vi "Main.vi"() -> ()   [LabVIEW 2014]
doc: "This template is for the Queued Message Handler design pattern.\n\nThe Event Handling Loop generates messages based on user interface actions.\n\nThe Message Handling Loop processes messages generated by the Event Handling Loop, or by other messages. The messages are string values, so new messages can be added easily to the Message Cases case structure in the Message Handling Loop. Each message cluster can also provide an optional value for Message Data, which is a variant that can be converted to whatever message-specific data is required."
uses:
  support/Type Definitions/UI Data.ctl
  support/Message Queue/Message Queue.lvlib
  Support/User Event - EHL Stop/User Event - EHL Stop.lvlib
  support/Message Queue/Enqueue Message (Single).vi
  <vilib>/ErrorRing/Error Ring.xnode
  Model/Model.lvlib
  DAQ/DAQ.lvlib
  DAQ/TypeDefs/DAQ data.ctl
  PLC/PLC.lvlib
  Logger/Logger.lvlib
  support/Status Logger/Status Log.ctl
  TCP/TCP.lvlib
  TCP/TypeDefs/TCP Data.ctl
  support/Global names.vi
  <vilib>/Utility/error.llb/DialogType.ctl
  <vilib>/Utility/error.llb/Error Cluster From Error Code.vi
  Report/Report.lvlib
  Report/TypeDefs/Report state.ctl
panel:
  out "Power status":bool
  in  "Remote":bool
  in  "Abort":bool
  in  "Stop Line":bool
  in  "Start Line":bool
  out "Status":string
  in  "Tab Control":T1(tab)
  in  "Power switch":bool
  in  "Positon":dbl(slide) scale=0.0..20.0
  in  "Dispose":bool
  in  "Pump":bool
  in  "Flow [l/s]":dbl=10.0
  in  "Potentiometer (AI)":tag
  in  "LED (DO)":tag
  in  "Bistable switch (DI)":tag
  in  "Monostable switch (DI)":tag
  in  "Send":bool
  in  "Message to send":string
  out "Message received":string
  in  "Disconnect":bool
  in  "Connect":bool
  out "Connected?":bool
  in  "Type":enum16{"Server", "Client"}(ring)
  in  "Port":u16
  in  "IP":string
  out "Current machine IP":string
  in  "Current printer":u16(ring) items=["PDFCreator", "OKI DATA CORP C5950 kolor (C-2 218)", "Microsoft XPS Document Writer", "Microsoft Print to PDF", "HP LaserJet Professional P1606dn B&W (M3)", "hp LaserJet 1320 PCL 5 B&W (C-2 307)", "Fax", "Canon MP560 KOLOR (DOM)", "Brother PC-FAX v.3.2", "Brother MFC-L8850CDW KOLOR (M6)", "Brother MFC-L2740DW B&W (M6)", "Brother MFC-L2740DW B&W (M3)", "Brother DCP-9020CDW (Dziekan)"]
  in  "Check printers":bool
  in  "Print report":bool
  in  "TDMS View":bool
  in  "Exit":bool
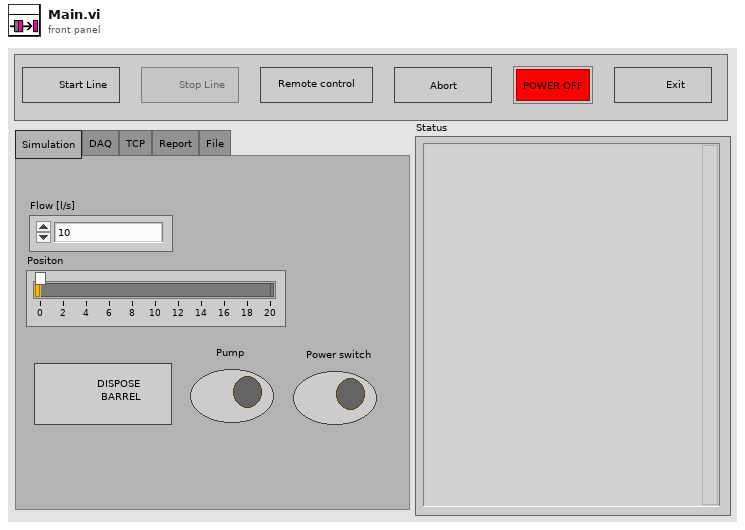
[diagram p1: front panel]
types:
  T1 = enum32{"Simulation", "DAQ", "TCP", "Report", "File"}
  T2 = typedef "Status Log.ctl" = enum16{"Close file", "Open Status file", "Add Status", "Show Status File"}
  T3 = typedef "UI Data.ctl" = cluster{"Start Line Ref":refnum<vi>, "Stop Line Ref":refnum<vi>, "Data Display Ref":refnum<vi>, "Exit Button Ref":refnum<vi>, "Pump Ref":refnum<vi>, "Dispose Ref":refnum<vi>, "Flow Ref":refnum<vi>, "Position Ref":refnum<vi>, "Tab Ref":refnum<vi>, "Print report":refnum<vi>, "Remote":refnum<vi>, "Connection status":refnum<vi>, "Abort":refnum<vi>, "Power status":refnum<vi>, "Power switch":refnum<vi>}
  T4 = typedef "Notifiers.lvlib/Notifiers.ctl" = cluster{"PLC":refnum<notifier>, "Model":refnum<notifier>, "DAQ":refnum<notifier>, "Log":refnum<notifier>, "TCP":refnum<notifier>}
  T5 = typedef "Message Queue.lvlib/All Message Queues.ctl" = cluster{"UI":refnum<queue>, "Model":refnum<queue>, "DAQ":refnum<queue>, "PLC":refnum<queue>, "Log":refnum<queue>, "TCP":refnum<queue>}
  T6 = typedef "Report.lvlib/Report state.ctl" = enum16{"Create report", "Save data", "Save report", "Available printers", "Print report", "Close report"}
  T7 = typedef "TCP.lvlib/TCP Data.ctl" = cluster{"Type":enum16{"Server", "Client"}, "IP":string, "Port":u16, "connection ID":refnum<k5>, "Connected?":bool, "Data":string}
  T8 = typedef "DialogType.ctl" = u16
  T9 = typedef "DAQ.lvlib/DAQ data.ctl" = cluster{"Power switch (DI)":cluster{"Channel":tag, "Data":bool}, "Dispose barrel (DI)":cluster{"Channel":tag, "Data":bool}, "Pump status (DO)":cluster{"Channel":tag, "Data":bool}, "Barrel position (AI)":cluster{"Channel":tag, "Data":dbl}}
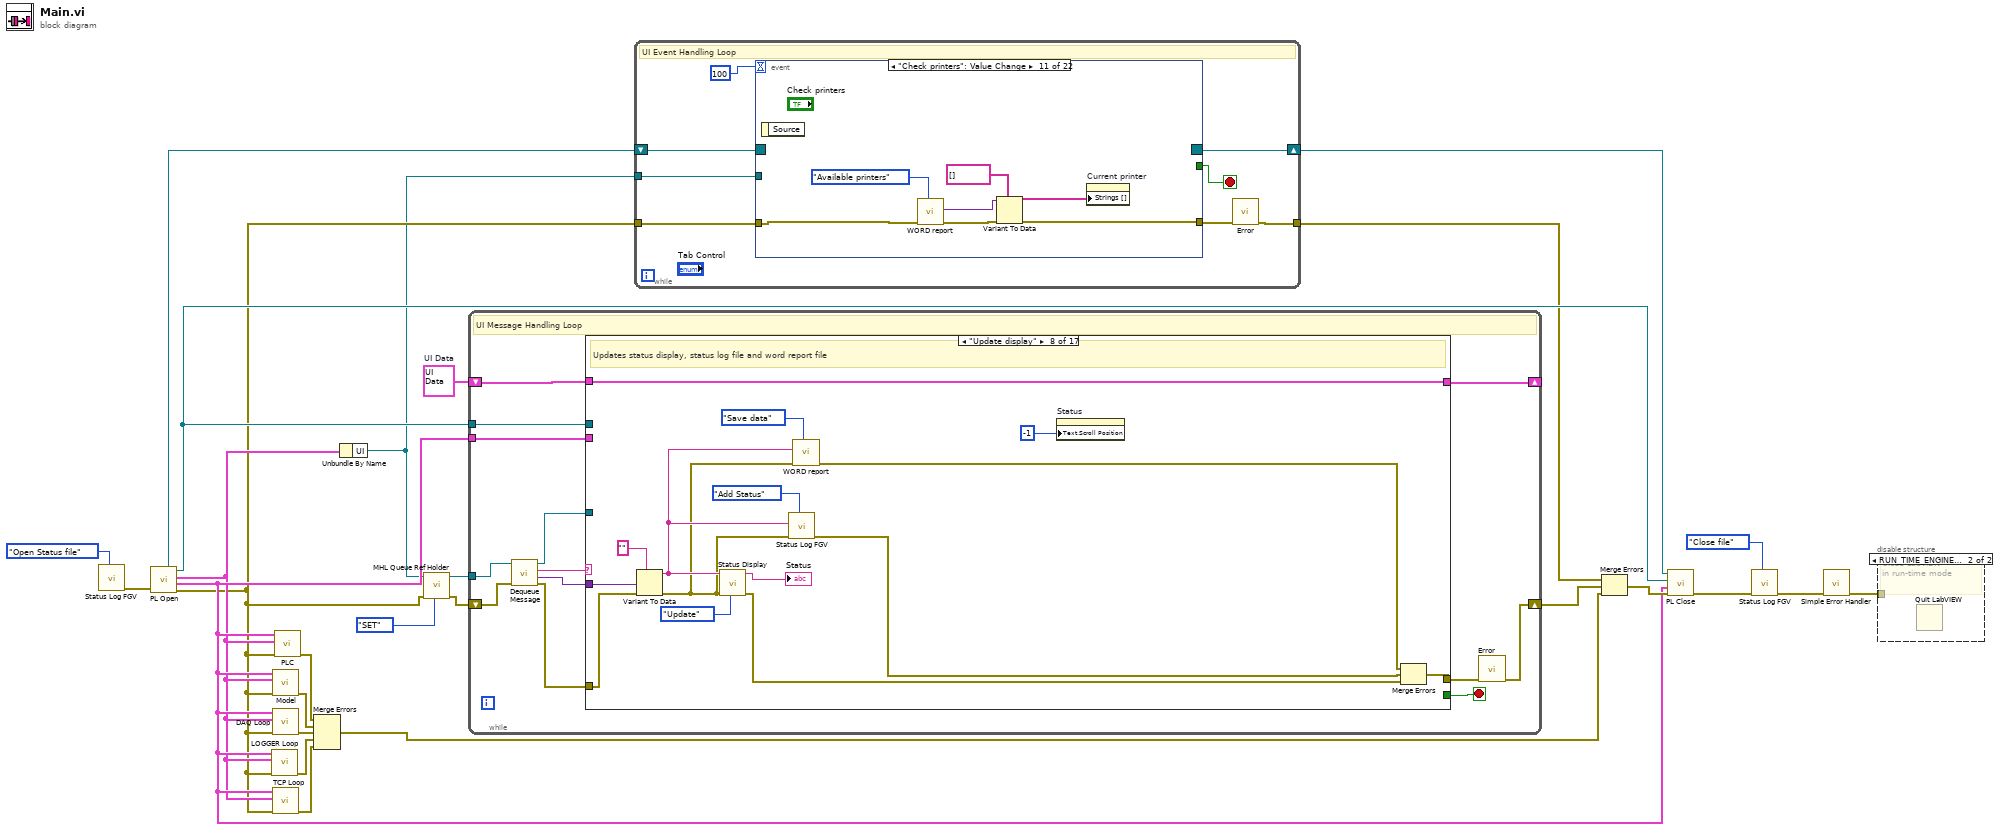
[diagram p0: block diagram]
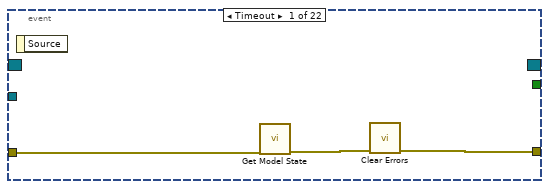
[diagram p2: hidden frame]
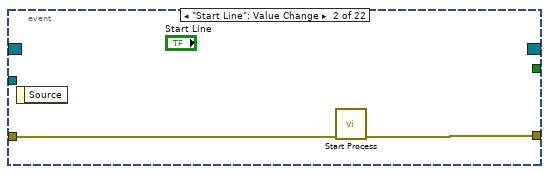
[diagram p3: hidden frame]
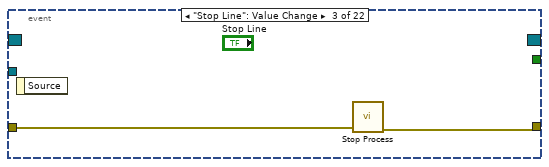
[diagram p4: hidden frame]
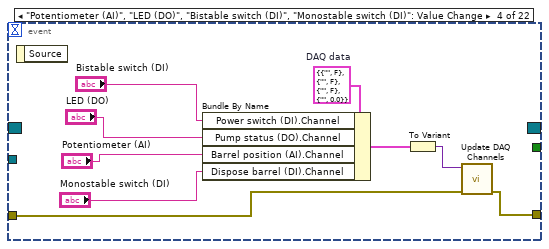
[diagram p5: hidden frame]
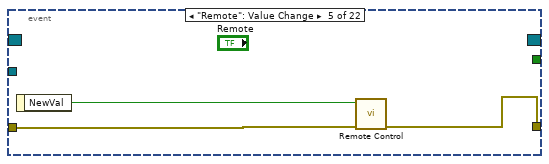
[diagram p6: hidden frame]
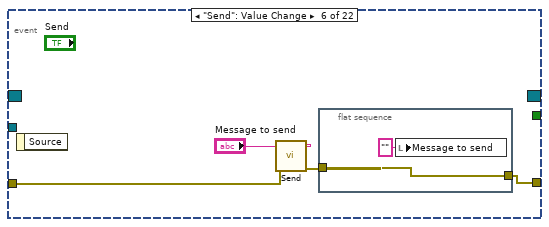
[diagram p7: hidden frame]
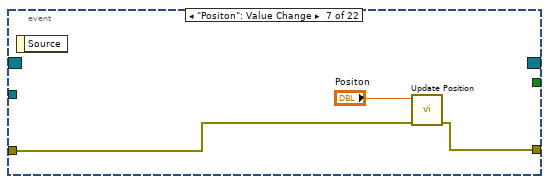
[diagram p8: hidden frame]
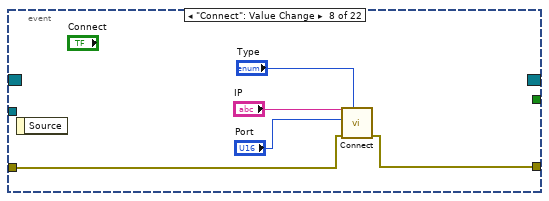
[diagram p9: hidden frame]
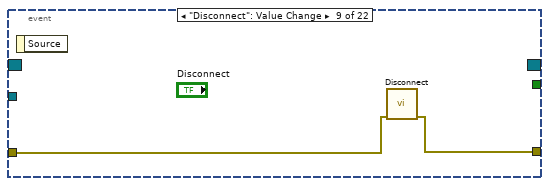
[diagram p10: hidden frame]
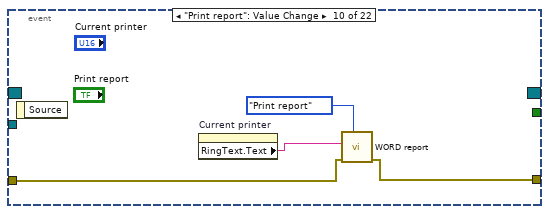
[diagram p11: hidden frame]
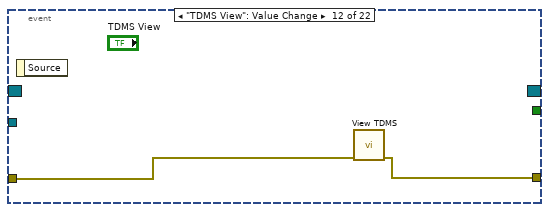
[diagram p12: hidden frame]
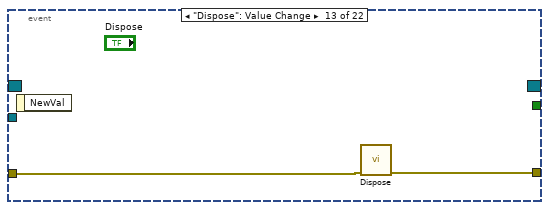
[diagram p13: hidden frame]
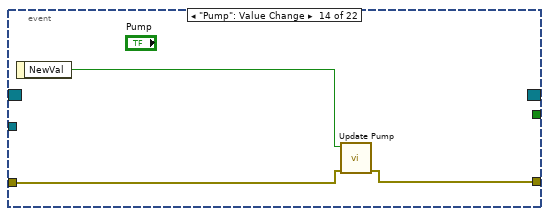
[diagram p14: hidden frame]
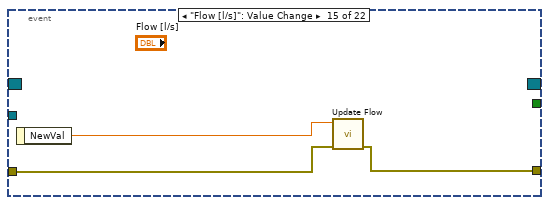
[diagram p15: hidden frame]
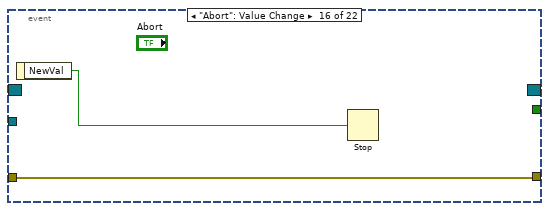
[diagram p16: hidden frame]
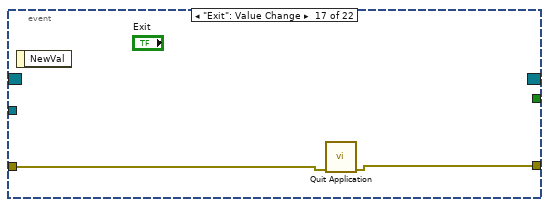
[diagram p17: hidden frame]
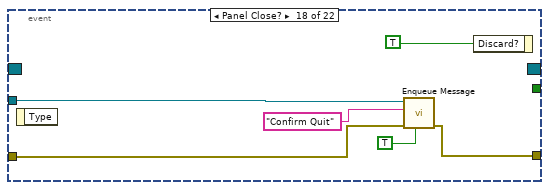
[diagram p18: hidden frame]
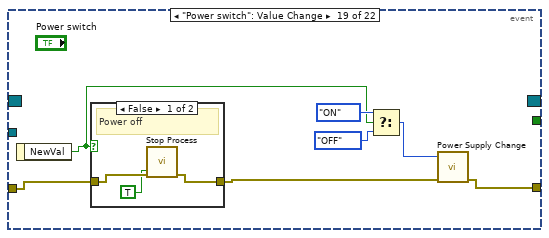
[diagram p19: hidden frame]
diagram:
  w25 = T3 {"Start Line Ref"=refnum, "Stop Line Ref"=refnum, "Data Display Ref"=refnum, "Exit Button Ref"=refnum, "Pump Ref"=refnum, "Dispose Ref"=refnum, "Flow Ref"=refnum, "Position Ref"=refnum, "Tab Ref"=refnum, "Print report"=refnum, "Remote"=refnum, "Connection status"=refnum, "Abort"=refnum, "Power status"=refnum, "Power switch"=refnum}  # UI Data
  n1 = call "Status Log FGV.vi"("Action"=Status_Log."Open Status file") -> ("error out"=w20:errorcluster)  [unwired: 10 in]
  n2 = call "PL Open.vi"("error in"=w20) -> ("error out"=w4:errorcluster, "Notifiers"=w13:T4, "Queues"=w12:T5, "User Event"=w23:refnum<user-event>, "Event Registration Refnum"=w15:refnum<event-registration>)  [unwired: 6 in]
  n3 = call "LOGGER Loop.vi"("error in"=w4, "Queues"=w12, "Notifiers"=w13) -> ("error out"=w8:errorcluster)  [unwired: 8 in]
  n4 = call "Model.vi"("error in"=w4, "Queues"=w12, "Notifiers"=w13) -> ("error out"=w10:errorcluster)  [unwired: 8 in]
  n5 = call "DAQ Loop.vi"("error in"=w4, "Queues"=w12, "Notifiers"=w13) -> ("error out"=w9:errorcluster)  [unwired: 8 in]
  n6 = call "TCP Loop.vi"("error in"=w4, "Queues"=w12, "Notifiers"=w13) -> ("error out"=w7:errorcluster)  [unwired: 8 in]
  n7 = call "PLC.vi"("error in"=w4, "Message Queues"=w12, "Notifiers"=w13) -> ("error out"=w11:errorcluster)  [unwired: 8 in]
  n8 = Merge Errors(w11, w10, w9, w8, w7) -> (w6:errorcluster)
  n9 = Unbundle By Name(w12) -> ("UI"=w1:refnum<queue>)
  n10 = call "MHL Queue Ref Holder.vi"("Action"=enum16{"GET", "SET"}."SET", "error in"=w4, "Message Queue In"=w1) -> ("error out"=w3:errorcluster, "Input Message Queue"=w5:refnum<queue>)  [unwired: 7 in]
  n11 = while {
    shift-right: [w38] -> _
    shift-left: w25 -> [w39]
    tunnel: w23 -> [w36]
    tunnel: w13 -> [w32]
    shift-right: [w28] -> w19
    shift-left: w3 -> [w35]
    tunnel: w5 -> [w30]
    stop <- w37 stop-if-true
    # "UI Message Handling Loop"
    n12 = call "Dequeue Message.vi"("error in (no error)"=w35, "Message Queue"=w30) -> ("error out"=w34:errorcluster, "Message Data"=w31:variant, "Message"=w27:string, "dup Message Queue"=w33:refnum<queue>)  [unwired: 6 in]
    n13 = case "Message Cases" shown="\"Update display\"" w27 {
      selector: w27 -> [_ _ _ _ _ _ _ _ _ _ _ _ _ _ _ _ w285]
      tunnel: w33 -> [w41 _ _ _ _ _ _ _ _ _ _ _ w231 w237 w273 _ _]
      tunnel: w34 -> [w42 w48 w71 w106 w112 w142 w160 w163 w180 w192 w220 w223 w232 w239 w256 w280 _]
      tunnel: [w40 w48 w81 w107 w124 w144 w156 w166 w181 w186 w216 w222 w229 w236 w260 w274 w284] -> w29
      tunnel: w39 -> [w43 w62 w92 w108 w129 w154 w155 w171 w184 w185 w198 w227 w233 w243 w265 w279 w286]
      tunnel: [w43 w49 w92 w108 w129 w154 w155 w171 w184 w185 w198 w227 w233 w243 w265 w279 w286] -> w38
      tunnel: [_ _ _ _ _ _ _ _ _ _ _ _ _ _ TRUE _ _] -> w37
      tunnel: w31 -> [_ _ _ _ _ _ w159 w175 w178 w191 w219 w226 _ _ w267 _ _]
      tunnel: w36 -> [_ _ _ _ _ _ _ _ _ _ _ _ _ _ w270 _ _]
      tunnel: w32 -> [_ _ _ _ _ _ _ _ _ _ _ _ _ w242 _ _ _]
      frame "Initialize" {
        w44 = string[] ["Initialize references", "Initialize controls", "Initialize PLC"]  # Message
        # "Prepare application initialization procedure"
        n14 = call "Enqueue Message (Array).vi"("error in (no error)"=w42, "Message Array"=w44, "Message Queue"=w41) -> ("error out"=w40:errorcluster)  [unwired: 7 in, 1 out]
      }
      frame "Initialize references" {
        # "Link references to UI objects"
        n15 = control-ref of="Power switch"() -> (w45:refnum<vi>)
        n16 = control-ref of="Stop Line"() -> (w59:refnum<vi>)
        n17 = control-ref of="Flow [l/s]"() -> (w56:refnum<vi>)
        n18 = control-ref of="Dispose"() -> (w57:refnum<vi>)
        n19 = control-ref of="Exit"() -> (w61:refnum<vi>)
        n20 = control-ref of="Start Line"() -> (w60:refnum<vi>)
        n21 = control-ref of="Pump"() -> (w58:refnum<vi>)
        n22 = Bundle By Name(cluster=w62, "Exit Button Ref"=w61, "Start Line Ref"=w60, "Stop Line Ref"=w59, "Pump Ref"=w58, "Dispose Ref"=w57, "Flow Ref"=w56, "Power switch"=w45) -> (w55:T3)
        n23 = control-ref of="Tab Control"() -> (w53:refnum<vi>)
        n24 = control-ref of="Remote"() -> (w51:refnum<vi>)
        n25 = control-ref of="Connection status"() -> (w50:refnum<vi>)
        n26 = control-ref of="Positon"() -> (w54:refnum<vi>)
        n27 = control-ref of="Print report"() -> (w52:refnum<vi>)
        n28 = control-ref of="Power status"() -> (w46:refnum<vi>)
        n29 = control-ref of="Abort"() -> (w47:refnum<vi>)
        n30 = Bundle By Name(cluster=w55, "Position Ref"=w54, "Tab Ref"=w53, "Print report"=w52, "Remote"=w51, "Connection status"=w50, "Abort"=w47, "Power status"=w46) -> (w49:T3)
      }
      frame "Initialize controls" {
        w80 = "" ("Data received")
        w63 = TRUE ("Enabled")
        w64 = FALSE ("Enabled")
        # "Initialize activity and values of UI objects"
        n31 = Unbundle By Name(w92) -> ("Stop Line Ref"=w105:refnum<vi>, "Print report"=w87:refnum<vi>)
        n32 = Current VI's Menubar() -> (w66:refnum<k9>)
        n33 = Build Array(w105, w87) -> (w104:refnum<vi>[])
        n34 = call "Enable Multiple Controls.vi"("error in"=w71, "Enabled"=w64, "References"=w104) -> ("error out"=w101:errorcluster)  [unwired: 8 in]
        n35 = Set Menu Item Info(7:"Stop" ("item tag"), 8:w71, 9:w64, 11:w66) -> (0:w69:errorcluster, 3:w65:refnum<k9>)  [unwired: 3 in]
        n36 = Unbundle By Name(w92) -> ("Exit Button Ref"=w103:refnum<vi>, "Start Line Ref"=w102:refnum<vi>)
        n37 = call "Power Supply Change.vi"("error in"=w71, "Power status"=enum16{"OFF", "ON"}."OFF") -> ("error out"=w77:errorcluster)  [unwired: 9 in]
        n38 = Build Array(w103, w102) -> (w100:refnum<vi>[])
        n39 = call "Enable Multiple Controls.vi"("error in"=w101, "Enabled"=w63, "References"=w100) -> ("error out"=w95:errorcluster)  [unwired: 8 in]
        n40 = Set Menu Item Info(7:"Start" ("item tag"), 8:w69, 9:w63, 11:w65) -> (0:w67:errorcluster)  [unwired: 3 in, 1 out]
        n41 = Unbundle By Name(w92) -> ("Exit Button Ref"=w99:refnum<vi>, "Start Line Ref"=w98:refnum<vi>, "Stop Line Ref"=w97:refnum<vi>, "Pump Ref"=w96:refnum<vi>, "Remote"=w86:refnum<vi>, "Connection status"=w85:refnum<vi>, "Abort"=w84:refnum<vi>, "Power status"=w83:refnum<vi>, "Power switch"=w73:refnum<vi>)
        n42 = call "Status Display.vi"("Action"=enum16{"Update", "Clear"}."Clear", "error in"=w77) -> ("error out"=w76:errorcluster, "Status"=w74:string)  [unwired: 8 in]
        n43 = local write "Status"(w74) -> ()
        n44 = Build Array(w99, w98, w97, w96, w86, w85, w84, w83, w73) -> (w93:refnum<vi>[])
        n45 = call "Value Multiple Boolean Controls.vi"("error in"=w95, "Value"=FALSE ("Enabled"), "References"=w93) -> ("error out"=w91:errorcluster)  [unwired: 8 in]
        n46 = Unbundle By Name(w92) -> ("Position Ref"=w90:refnum<vi>)
        n47 = Build Array(w90) -> (w89:refnum<vi>[])
        n48 = call "Value Multiple Numeric Controls.vi"("error in"=w91, "Value"=0.0, "References"=w89) -> ("error out"=w79:errorcluster)  [unwired: 8 in]
        n49 = local write "Message received"(w80) -> ()
        n50 = local write "Message to send"(w80) -> ()
        n51 = call "Update Display.vi"("error in"=w79, "Message string"="UI initialized") -> ("error out"=w68:errorcluster)  [unwired: 9 in]
        n52 = Merge Errors(w68, w67, w76) -> (w81:errorcluster)
      }
      frame "Initialize PLC" {
        # "Initialize Production Line Controller"
        n53 = call "Initialize.vi"("error in"=w106) -> ("error out"=w107:errorcluster)  [unwired: 10 in]
      }
      frame "Start process" {
        w116 = TRUE ("Enabled")
        w120 = FALSE ("Enabled")
        # "Starts process: start PLC, open logger file, create reports files, enable/disable UI controls and update status display"
        n54 = Unbundle By Name(w129) -> ("Exit Button Ref"=w113:refnum<vi>, "Start Line Ref"=w125:refnum<vi>, "Stop Line Ref"=w128:refnum<vi>)
        n55 = Build Array(w113, w125) -> (w130:refnum<vi>[])
        n56 = Build Array(w128) -> (w127:refnum<vi>[])
        n57 = call "Start.vi"("error in"=w112) -> ("error out"=w126:errorcluster)  [unwired: 10 in]
        n58 = call "WORD report.vi"("Action"=Report_state."Create report", "error in"=w112) -> ("error out"=w110:errorcluster)  [unwired: 8 in, 1 out]
        n59 = call "Enable Multiple Controls.vi"("error in"=w112, "Enabled"=w116, "References"=w127) -> ("error out"=w118:errorcluster)  [unwired: 8 in]
        n60 = call "Enable Multiple Controls.vi"("error in"=w112, "Enabled"=w120, "References"=w130) -> ("error out"=w122:errorcluster)  [unwired: 8 in]
        n61 = global read "Global names.vi" "Starting"() -> (w114:string)
        n62 = Current VI's Menubar() -> (w115:refnum<k9>)
        n63 = call "Update Display.vi"("error in"=w126, "Message string"=w114) -> ("error out"=w111:errorcluster)  [unwired: 9 in]
        n64 = Set Menu Item Info(7:"Start" ("item tag"), 8:w122, 9:w120, 11:w115) -> (0:w121:errorcluster)  [unwired: 3 in, 1 out]
        n65 = Set Menu Item Info(7:"Stop" ("item tag"), 8:w118, 9:w116, 11:w115) -> (0:w117:errorcluster)  [unwired: 3 in, 1 out]
        n66 = Merge Errors(w111, w110, w121, w117) -> (w124:errorcluster)
      }
      frame "Stop process" {
        w133 = FALSE ("Enabled")
        w134 = TRUE ("Enabled")
        # "Stops process: stop PLC, close logger file, save and close report files, enable/disable UI controls and update status display"
        n67 = Unbundle By Name(w154) -> ("Exit Button Ref"=w131:refnum<vi>, "Start Line Ref"=w147:refnum<vi>, "Stop Line Ref"=w153:refnum<vi>)
        n68 = call "Stop.vi"("error in"=w142) -> ("error out"=w149:errorcluster)  [unwired: 10 in]
        n69 = Build Array(w153) -> (w143:refnum<vi>[])
        n70 = Build Array(w131, w147) -> (w151:refnum<vi>[])
        n71 = global read "Global names.vi" "Stopping"() -> (w132:string)
        n72 = Build Array (concatenate)(w151, w143) -> (w150:refnum<vi>[])
        n73 = call "Enable Multiple Controls.vi"("error in"=w142, "Enabled"=w134, "References"=w151) -> ("error out"=w139:errorcluster)  [unwired: 8 in]
        n74 = call "Enable Multiple Controls.vi"("error in"=w142, "Enabled"=w133, "References"=w143) -> ("error out"=w146:errorcluster)  [unwired: 8 in]
        n75 = call "Value Multiple Boolean Controls.vi"("error in"=w142, "Value"=FALSE, "References"=w150) -> ("error out"=w145:errorcluster)  [unwired: 8 in]
        n76 = call "Update Display.vi"("error in"=w149, "Message string"=w132) -> ("error out"=w148:errorcluster)  [unwired: 9 in]
        n77 = Current VI's Menubar() -> (w140:refnum<k9>)
        n78 = Set Menu Item Info(7:"Start" ("item tag"), 8:w139, 9:w134, 11:w140) -> (0:w137:errorcluster, 3:w135:refnum<k9>)  [unwired: 3 in]
        n79 = Set Menu Item Info(7:"Stop" ("item tag"), 8:w137, 9:w133, 11:w135) -> (0:w136:errorcluster)  [unwired: 3 in, 1 out]
        n80 = Merge Errors(w148, w136, w146, w145) -> (w144:errorcluster)
      }
      frame "Update IP" {
        # "Update IP address of current machine"
        n81 = Variant To Data(error in=w160, type="", Variant=w159) -> (data=→"Current machine IP":string, error out=w156:errorcluster)
      }
      frame "Update display" {
        # "Updates status display, status log file and word report file"
        n82 = Variant To Data(error in=w163, type="", Variant=w175) -> (data=w165:string, error out=w162:errorcluster)
        n83 = call "Status Display.vi"("Action"=enum16{"Update", "Clear"}."Update", "error in"=w162, "Status line"=w165) -> ("error out"=w167:errorcluster, "Status"=→"Status":string)  [unwired: 7 in]
        n84 = call "Status Log FGV.vi"("Action"=Status_Log."Add Status", "error in"=w162, "Status"=w165) -> ("error out"=w168:errorcluster)  [unwired: 8 in]
        n85 = call "WORD report.vi"("Action"=Report_state."Save data", "error in"=w162, "Data in"=w165) -> ("error out"=w161:errorcluster)  [unwired: 7 in, 1 out]
        n86 = property on="Status" class="Str"("Text.Scroll Position"=-1) -> ()  [unwired: 2 in, 2 out]
        n87 = Merge Errors(w161, w168, w167) -> (w166:errorcluster)
      }
      frame "Update position" {
        # "Programmatically update position of the barrel slider"
        n88 = Variant To Data(error in=w180, type=0.0 ("Value"), Variant=w178) -> (data=w176:dbl, error out=w179:errorcluster)
        n89 = Unbundle By Name(w184) -> ("Position Ref"=w183:refnum<vi>)
        n90 = Build Array(w183) -> (w182:refnum<vi>[])
        n91 = call "Value Multiple Numeric Controls.vi"("error in"=w179, "Value"=w176, "References"=w182) -> ("error out"=w181:errorcluster)  [unwired: 8 in]
      }
      frame "Update Connection UI" {
        w190 = T7 {"Type"=enum."Server", "IP"="", "Port"=0, "connection ID"=refnum, "Connected?"=FALSE, "Data"=""}  # TCP Data
        # "Updates TCP conection UI indicators"
        n92 = Variant To Data(error in=w192, type=w190, Variant=w191) -> (data=w189:T7, error out=w186:errorcluster)
        n93 = Unbundle By Name(w189) -> ("Connected?"=→"Connected?":bool, "Data"=→"Message received":string)
      }
      frame "Power status change" {
        # "Update main switch LED and Start/Stop buttons according to power status change (DAQ DI)"
        n94 = Variant To Data(error in=w220, type=TRUE, Variant=w219) -> (data=w199:bool, error out=w203:errorcluster)
        "Power status" <- w199
        n95 = Unbundle By Name(w198) -> ("Position Ref"=w193:refnum<vi>, "Dispose Ref"=w197:refnum<vi>, "Pump Ref"=w196:refnum<vi>)
        n96 = Unbundle By Name(w198) -> ("Start Line Ref"=w195:refnum<vi>, "Stop Line Ref"=w217:refnum<vi>)
        n97 = Build Array(w193, w197, w196, w195) -> (w194:refnum<vi>[])
        n98 = Build Array(w195) -> (w215:refnum<vi>[])
        n99 = Build Array(w217) -> (w212:refnum<vi>[])
        n100 = Build Array (concatenate)(w215, w212) -> (w214:refnum<vi>[])
        n101 = Current VI's Menubar() -> (w206:refnum<k9>)
        n102 = call "Enable Multiple Controls.vi"("error in"=w203, "Enabled"=w199, "References"=w194) -> ("error out"=w210:errorcluster)  [unwired: 8 in]
        n103 = Set Menu Item Info(7:"Start" ("item tag"), 8:w203, 9:w199, 11:w206) -> (0:w204:errorcluster, 3:w200:refnum<k9>)  [unwired: 3 in]
        n104 = call "Value Multiple Boolean Controls.vi"("error in"=w203, "Value"=FALSE, "References"=w214) -> ("error out"=w209:errorcluster)  [unwired: 8 in]
        n105 = call "Enable Multiple Controls.vi"("error in"=w203, "Enabled"=FALSE, "References"=w212) -> ("error out"=w208:errorcluster)  [unwired: 8 in]
        n106 = Set Menu Item Info(7:"Stop" ("item tag"), 8:w204, 9:FALSE ("enabled"), 11:w200) -> (0:w201:errorcluster)  [unwired: 3 in, 1 out]
        n107 = Merge Errors(w210, w209, w208, w201) -> (w216:errorcluster)
      }
      frame "Error" {
        w221 = T8 2 items=["no dialog", "OK message", "continue or stop message", "OK message + warnings", "continue/stop + warnings"] ("type of dialog (OK msg:1)")
        # "Display error dialog box and quit application"
        n108 = Variant To Data(error in=w223, type=errorcluster {"status"=FALSE, "code"=0, "source"=""} ("error constant"), Variant=w226) -> (data=w224:errorcluster, error out=w222:errorcluster)
        n109 = call <vilib>:"Simple Error Handler.vi"("type of dialog (OK msg:1)"=w221, "error in (no error)"=w224) -> ()  [unwired: 3 in, 5 out]
      }
      frame "Exit" {
        # "Start exit procedure: stop PLC, then send Exit message to PLC and go to PLC confirmation loop"
        n110 = Flush Queue(queue=w231, error in (no error)=w232) -> (error out=w228:errorcluster)  [unwired: 2 out]
        n111 = call "Exit PLC.vi"("error in"=w228) -> ("error out"=w230:errorcluster)  [unwired: 10 in]
        n112 = call "Wait on PLC Exit.vi"("error in"=w230) -> ("error out"=w229:errorcluster)  [unwired: 10 in]
      }
      frame "Wait on PLC exit" {
        # "Wait until PLC shutdown"
        n113 = Unbundle By Name(w242) -> ("PLC"=w241:refnum<notifier>)
        n114 = Wait on Notification(notifier=w241, timeout in ms (-1)=10, error in (no error)=w239) -> (notification=w235:string, timed out?=w238:bool, error out=w234:errorcluster)  [unwired: 1 in, 1 out]
        n115 = case shown="True" w238 {
          tunnel: [w244 w253] -> w236
          tunnel: w234 -> [w245 w250]
          tunnel: w237 -> [_ w251]
          tunnel: w235 -> [_ w246]
          frame True {
            # "Shutdown notification from PLC not received"
            n116 = call "Wait on PLC Exit.vi"("error in"=w245) -> ("error out"=w244:errorcluster)  [unwired: 10 in]
          }
          frame False {
            # "Shutdown notification from PLC received (handshake)"
            n117 = call "Update Display.vi"("error in"=w250, "Message string"=w246) -> ("error out"=w249:errorcluster)  [unwired: 9 in]
            n118 = call "Update Display.vi"("error in"=w249, "Message string"="Application quits" ("Message")) -> ("error out"=w248:errorcluster)  [unwired: 9 in]
            n119 = call-poly "Enqueue Message.vi"("error in (no error)"=w248, "Message"="End program", "Message Queue"=w251) -> ("error out"=w253:errorcluster)  [unwired: 7 in, 1 out]
          }
        }
      }
      frame "End program" {
        # "Shutdown MHL and send exit user event to EHL; reset UI controls"
        n120 = call "Fire User Event - EHL Stop.vi"("error in (no error)"=w256, "User Event - Stop"=w270) -> ("error out"=w255:errorcluster)  [unwired: 9 in]
        n121 = Variant To Data(error in=w256, type=errorcluster {"status"=FALSE, "code"=0, "source"=""} ("error constant"), Variant=w267) -> (data=w268:errorcluster)  [unwired: 1 out]
        n122 = Release Queue(queue=w273, force destroy? (F)=TRUE, error in (no error)=w256) -> (error out=w271:errorcluster)  [unwired: 2 out]
        n123 = call <vilib>:"Simple Error Handler.vi"("error in (no error)"=w268) -> ("error out"=w254:errorcluster)  [unwired: 4 in, 4 out]
        n124 = Merge Errors(w255, w254, w271) -> (w261:errorcluster)
        n125 = Unbundle By Name(w265) -> ("Exit Button Ref"=w264:refnum<vi>, "Abort"=w259:refnum<vi>, "Start Line Ref"=w258:refnum<vi>, "Stop Line Ref"=w257:refnum<vi>)
        n126 = Build Array(w264, w259, w258, w257) -> (w263:refnum<vi>[])
        n127 = call "Value Multiple Boolean Controls.vi"("error in"=w261, "Value"=FALSE, "References"=w263) -> ("error out"=w260:errorcluster)  [unwired: 8 in]
      }
      frame "Confirm Quit" {
        # "Confirm Quit - Message that can confirm whether or not the user wants to exit the application."
        n128 = Two Button Dialog(message="Are you sure?", 1:"Continue" ("F button name (\"Cancel\")"), 2:"Quit" ("T button name (\"OK\")")) -> (T button?=w275:bool)
        n129 = case shown="True" w275 {
          tunnel: w280 -> [w281 w283]
          tunnel: [w281 w282] -> w274
          frame False {
          }
          frame True {
            n130 = call "Quit Application.vi"("error in"=w283) -> ("error out"=w282:errorcluster)  [unwired: 10 in]
          }
        }
      }
      frame Default {
        # "Incorrect message: show error and clear error"
        n131 = xnode "Error Ring"("parameter 0"=w285) -> ("error out"=w284:errorcluster)
      }
    }
    n132 = call "Error.vi"("error in"=w29) -> ("error out"=w28:errorcluster)  [unwired: 10 in]
  }
  n133 = while {
    tunnel: w1 -> [w296]
    shift-right: [w300] -> w26
    shift-left: w15 -> [w301]
    tunnel: [w294] -> w14
    tunnel: w4 -> [w297]
    stop <- w299 stop-if-true
    # "UI Event Handling Loop"
    n134 = event shown="[10] \"Check printers\": Value Change" {
      selector: w301 -> [_ _ _ _ _ _ _ _ _ _ _ _ _ _ _ _ _ _ _ _ _ _]
      dyn-events: [_ _ _ _ _ _ _ _ _ _ _ _ _ _ _ _ _ _ _ _ _ _] -> w300
      timeout: 100 -> [_ _ _ _ _ _ _ _ _ _ _ _ _ _ _ _ _ _ _ _ _ _]
      tunnel: [_ _ _ _ _ _ _ _ _ _ _ _ _ _ _ _ _ _ _ _ TRUE ("Discard?") _] -> w299
      tunnel: w296 -> [_ _ _ _ _ _ _ _ _ _ _ _ _ _ _ _ _ w367 _ _ _ _]
      tunnel: [w302 w305 w307 w317 w320 w321 w328 w330 w335 w339 w344 w348 w350 w353 w356 w359 w360 w366 w368 w379 w380 w383] -> w295
      tunnel: w297 -> [w304 w306 w308 w316 w319 w322 w327 w331 w336 w340 w347 w349 w351 w354 w357 w359 w361 w362 w370 w379 w380 w382]
      event Timeout {
        n135 = event-data() -> ()  [unwired: 1 in, 1 out]
        n136 = call "Get Model State.vi"("error in (no error)"=w304) -> ("error out"=w303:errorcluster)  [unwired: 10 in]
        n137 = call <vilib>:"Clear Errors.vi"("error in (no error)"=w303) -> ("error out"=w302:errorcluster)  [unwired: 5 in, 1 out]
      }
      event "Start Line": Value Change {
        n138 = event-data() -> ()  [unwired: 1 in, 1 out]
        n139 = call "Start Process.vi"("error in"=w306) -> ("error out"=w305:errorcluster)  [unwired: 10 in]
      }
      event "Stop Line": Value Change {
        n140 = event-data() -> ()  [unwired: 1 in, 1 out]
        n141 = call "Stop Process.vi"("error in"=w308) -> ("error out"=w307:errorcluster)  [unwired: 10 in]
      }
      event "Potentiometer (AI)", "LED (DO)", "Bistable switch (DI)", "Monostable switch (DI)": Value Change {
        w310 = T9 {"Power switch (DI)"={"Channel"="", "Data"=FALSE}, "Dispose barrel (DI)"={"Channel"="", "Data"=FALSE}, "Pump status (DO)"={"Channel"="", "Data"=FALSE}, "Barrel position (AI)"={"Channel"="", "Data"=0.0}}  # DAQ data
        n142 = event-data() -> ()  [unwired: 1 in, 1 out]
        n143 = Bundle By Name(cluster=w310, "Power switch (DI).Channel"="Bistable switch (DI)", "Pump status (DO).Channel"="LED (DO)", "Barrel position (AI).Channel"="Potentiometer (AI)", "Dispose barrel (DI).Channel"="Monostable switch (DI)") -> (w313:T9)
        n144 = To Variant(anything=w313) -> (Variant=w309:variant)
        n145 = call "Update DAQ Channels.vi"("error in"=w316, "Message Data"=w309) -> ("error out"=w317:errorcluster)  [unwired: 9 in]
      }
      event "Remote": Value Change {
        n146 = event-data() -> ("NewVal"=w318:bool)  [unwired: 1 in]
        n147 = call "Remote Control.vi"("error in"=w319, "Remote"=w318) -> ("error out"=w320:errorcluster)  [unwired: 9 in]
      }
      event "Send": Value Change {
        n148 = event-data() -> ()  [unwired: 1 in, 1 out]
        n149 = call "Send.vi"("error in"=w322, "Data"="Message to send") -> ("error out"=w323:errorcluster)  [unwired: 9 in]
        n150 = flat-sequence {
          tunnel: w323 -> [w325]
          tunnel: [w325] -> w321
          frame #0 {
            n151 = local write "Message to send"("" ("Data to send")) -> ()
          }
        }
      }
      event "Positon": Value Change {
        n152 = event-data() -> ()  [unwired: 1 in, 1 out]
        n153 = call "Update Position.vi"("error in (no error)"=w327, "Position"="Positon") -> ("error out"=w328:errorcluster)  [unwired: 9 in]
      }
      event "Connect": Value Change {
        n154 = event-data() -> ()  [unwired: 1 in, 1 out]
        n155 = call "Connect.vi"("Type"="Type", "error in"=w331, "Port"="Port", "IP"="IP") -> ("error out"=w330:errorcluster)  [unwired: 7 in]
      }
      event "Disconnect": Value Change {
        n156 = event-data() -> ()  [unwired: 1 in, 1 out]
        n157 = call "Disconnect.vi"("error in"=w336) -> ("error out"=w335:errorcluster)  [unwired: 10 in]
      }
      event "Print report": Value Change {
        n158 = event-data() -> ()  [unwired: 1 in, 1 out]
        n159 = property on="Current printer" class="Ring (strict)"() -> ("RingText.Text"=w338:string)  [unwired: 2 in, 2 out]
        n160 = call "WORD report.vi"("Action"=Report_state."Print report", "error in"=w340, "Data in"=w338) -> ("error out"=w339:errorcluster)  [unwired: 7 in, 1 out]
      }
      event "Check printers": Value Change {
        n161 = event-data() -> ()  [unwired: 1 in, 1 out]
        n162 = call "WORD report.vi"("Action"=Report_state."Available printers", "error in"=w347) -> ("error out"=w345:errorcluster, "Data out"=w343:variant)  [unwired: 8 in]
        n163 = Variant To Data(error in=w345, type=string[] [], Variant=w343) -> (data=w341:string[], error out=w344:errorcluster)
        n164 = property on="Current printer" class="Ring (strict)"("Strings []"=w341) -> ()  [unwired: 2 in, 2 out]
      }
      event "TDMS View": Value Change {
        n165 = event-data() -> ()  [unwired: 1 in, 1 out]
        n166 = call "View TDMS.vi"("error in"=w349) -> ("error out"=w348:errorcluster)  [unwired: 10 in]
      }
      event "Dispose": Value Change {
        n167 = event-data() -> ()  [unwired: 1 in, 1 out]
        n168 = call "Dispose.vi"("error in (no error)"=w351) -> ("error out"=w350:errorcluster)  [unwired: 10 in]
      }
      event "Pump": Value Change {
        n169 = event-data() -> ("NewVal"=w352:bool)  [unwired: 1 in]
        n170 = call "Update Pump.vi"("error in (no error)"=w354, "Pump State"=w352) -> ("error out"=w353:errorcluster)  [unwired: 9 in]
      }
      event "Flow [l/s]": Value Change {
        n171 = event-data() -> ("NewVal"=w355:dbl)  [unwired: 1 in]
        n172 = call "Update Flow.vi"("error in (no error)"=w357, "Flow"=w355) -> ("error out"=w356:errorcluster)  [unwired: 9 in]
      }
      event "Abort": Value Change {
        n173 = event-data() -> ("NewVal"=w358:bool)  [unwired: 1 in]
        n174 = Stop(stop? (T)=w358) -> ()
      }
      event "Exit": Value Change {
        n175 = event-data() -> ()  [unwired: 1 in, 1 out]
        n176 = call "Quit Application.vi"("error in"=w361) -> ("error out"=w360:errorcluster)  [unwired: 10 in]
      }
      event Panel Close? {
        n177 = event-data() -> ()  [unwired: 1 in, 1 out]
        n178 = call-poly "Enqueue Message.vi"("Priority Message? (F)"=TRUE, "error in (no error)"=w362, "Message"="Confirm Quit", "Message Queue"=w367) -> ("error out"=w366:errorcluster)  [unwired: 6 in, 1 out]
        n179 = event-data("Discard?"=TRUE) -> ()  [unwired: 1 in, 1 out]
      }
      event "Power switch": Value Change {
        n180 = event-data() -> ("NewVal"=w371:bool)  [unwired: 1 in]
        n181 = case shown="False" w371 {
          tunnel: w370 -> [w377 w378]
          tunnel: [w376 w378] -> w369
          frame False {
            # "Power off"
            n182 = call "Stop Process.vi"("Priority Message? (F)"=TRUE, "error in"=w377) -> ("error out"=w376:errorcluster)  [unwired: 9 in]
          }
          frame True {
            # "Power on"
          }
        }
        n183 = Select(t=enum16{"OFF", "ON"}."ON" ("Power status"), s=w371, f=enum16{"OFF", "ON"}."OFF" ("Power status")) -> (s? t:f=w372:enum16{"OFF", "ON"})
        n184 = call "Power Supply Change.vi"("error in"=w369, "Power status"=w372) -> ("error out"=w368:errorcluster)  [unwired: 9 in]
      }
      event Application Instance Close {
        n185 = event-data() -> ()  [unwired: 1 in, 1 out]
      }
      event User Event {
        n186 = event-data() -> ()  [unwired: 1 in, 1 out]
      }
      event Menu Selection (User) {
        n187 = event-data() -> ("ItemTag"=w384:string)  [unwired: 1 in]
        n188 = case shown="\"logdir\"" w384 {
          tunnel: [w385 w388 w389 w393 w394 w396] -> w383
          tunnel: w382 -> [w385 w387 w390 w392 w395 w397]
          frame Default {
          }
          frame "logdir" {
            n189 = global read "Global names.vi" "Status log dir"() -> (w386:string)
            n190 = call "Open Dir.vi"("error in"=w387, "dir"=w386) -> ("error out"=w388:errorcluster)  [unwired: 9 in]
          }
          frame "statuslog" {
            n191 = call "Status Log FGV.vi"("Action"=Status_Log."Show Status File", "error in"=w390) -> ("error out"=w389:errorcluster)  [unwired: 9 in]
          }
          frame "Start" {
            n192 = call "Start Process.vi"("error in"=w392) -> ("error out"=w393:errorcluster)  [unwired: 10 in]
          }
          frame "Stop" {
            n193 = call "Stop Process.vi"("error in"=w395) -> ("error out"=w394:errorcluster)  [unwired: 10 in]
          }
          frame "Exit" {
            n194 = call "Quit Application.vi"("error in"=w397) -> ("error out"=w396:errorcluster)  [unwired: 10 in]
          }
        }
      }
    }
    n195 = call "Error.vi"("error in"=w295) -> ("error out"=w294:errorcluster)  [unwired: 10 in]
  }
  n196 = Merge Errors(w14, w19, w6) -> (w18:errorcluster)
  n197 = call "PL Close.vi"("error in"=w18, "Notifiers"=w13, "User Event"=w23, "Event Registration Refnum in"=w26) -> ("error out"=w24:errorcluster)  [unwired: 7 in]
  n198 = call "Status Log FGV.vi"("Action"=Status_Log."Close file", "error in"=w24) -> ("error out"=w16:errorcluster)  [unwired: 9 in]
  n199 = call <vilib>:"Simple Error Handler.vi"("error in (no error)"=w16) -> ("error out"=w17:errorcluster)  [unwired: 4 in, 4 out]
  n200 = disable-structure shown="RUN_TIME_ENGINE==True" {
    disable-tunnel: w17 -> [_ _]
    frame condition #0 (active) {
    }
    frame condition #1 {
      # "Close LabVIEW\nin run-time mode"
      n201 = Quit LabVIEW() -> ()  [unwired: 1 in]
    }
  }
